vi "Test Initialization.vi"() -> ()   [LabVIEW 2015, in "String Compare Tests.lvlib"]
uses:
  String Compare Tests.lvlib
  classes/Sequence/Config/Sequence Config.lvclass
  Config/String Compare Config.lvclass
  <vilib>/NI/Tag Bus/tag/Data Type.ctl
  <vilib>/NI/Tag Bus Module Framework/channel/channel classification.ctl
  Config/Mode.ctl
  Config/String Compare Config.lvclass/String Compare Config.ctl
  Config/Write Test Value Channel.vi
  Config/Write Result Channel.vi
  Config/Write Mode.vi
  Config/Write Limit_Regex.vi
  Config/Write ignore case.vi
  Config/Write Multiline.vi
  Config/Write offset.vi
  classes/Sequence/Execution/Sequence.lvclass
  <vilib>/NI/Tag Bus Module Framework/channel/TBM channel.lvclass
  <vilib>/NI/Tag Bus/tag/tag descriptor.lvclass
panel:
  out "error out":errorcluster
  out "Pass":bool
  out "Name":string
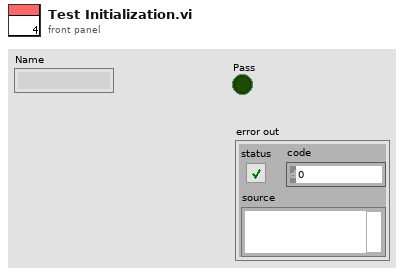
[diagram p1: front panel]
types:
  T1 = typedef "String Compare Config.lvclass/Mode.ctl" = enum16{"Compare Strings", "Match Regex"}
  T2 = typedef "TBM channel.lvclass/channel classification.ctl" = enum16{"input data", "output data", "processing parameter", "processing result"}
  T3 = typedef "tag bus.lvlib/tag descriptor.lvclass/Data Type.ctl" = enum16{"Double", "Single", "I64", "I32", "I16", "I8", "U64", "U32", "U16", "U8", "Boolean", "String", "Array of Double", "Array of Single", "Array of I64", "Array of I32", "Array of I16", "Array of I8", "Array of U64", "Array of U32", "Array of U16", "Array of U8", "Array of Boolean", "Array of String"}
  T4 = typedef "TBM channel.lvclass/data tables.ctl" = cluster{"input data":T5, "processing parameter":T5, "processing result":T5, "output data":T5}
  T5 = typedef "tag bus.lvlib/dictionary table pair.ctl" = cluster{"data dictionary":refnum<class "data dictionary.lvclass">, "data table":T6}
  T6 = typedef "tag bus.lvlib/data table.lvlib/data table.ctl" = cluster{"Double":dbl[], "Single":sgl[], "I64":i64[], "I32":i32[], "I16":i16[], "I8":i8[], "U64":u64[], "U32":u32[], "U16":u16[], "U8":u8[], "Boolean":bool[], "String":string[], "Array of Double":cluster{"DBL Array":dbl[]}[], "Array of Single":cluster{"SGL Array":sgl[]}[], "Array of I64":cluster{"I64 Array":i64[]}[], "Array of I32":cluster{"I32 Array":i32[]}[], "Array of I16":cluster{"I16 Array":i16[]}[], "Array of I8":cluster{"I8 Array":i8[]}[], "Array of U64":cluster{"U64 Array":u64[]}[], "Array of U32":cluster{"U32 Array":u32[]}[], "Array of U16":cluster{"U16 Array":u16[]}[], "Array of U8":cluster{"U8 Array":u8[]}[], "Array of Boolean":cluster{"Boolean Array":bool[]}[], "Array of String":cluster{"String Array":string[]}[]}
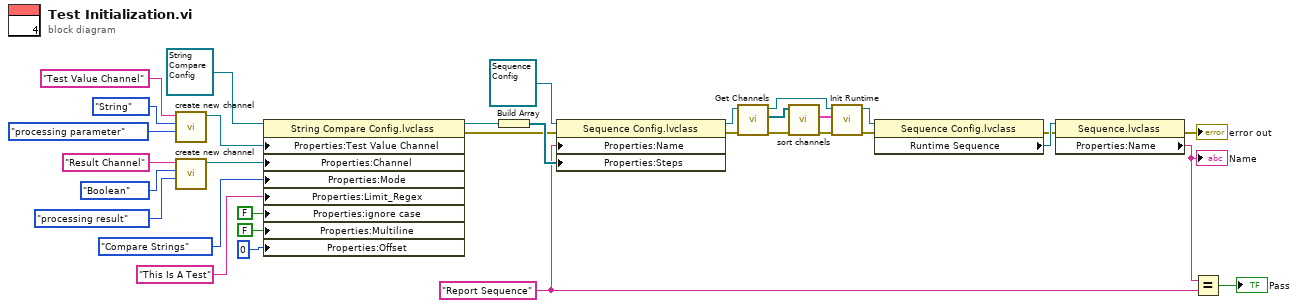
[diagram p0: block diagram]
diagram:
  w19 = "Report Sequence" ("Name")
  n1 = call <vilib>:"create new channel.vi"("channel classification"=channel_classification."processing parameter", "data type"=Data_Type."String", "channel name"="Test Value Channel") -> ("channel"=w9:refnum<class "TBM channel.lvclass">)  [unwired: 8 in]
  n2 = call <vilib>:"create new channel.vi"("channel classification"=channel_classification."processing result", "data type"=Data_Type."Boolean", "channel name"="Result Channel") -> ("channel"=w8:refnum<class "TBM channel.lvclass">)  [unwired: 8 in]
  n3 = property class="String Compare Config.lvclass"(reference=refnum<class "String Compare Config.lvclass"> refnum ("String Compare Config.lvclass"), "Properties:Test Value Channel"=w9, "Properties:Channel"=w8, "Properties:Mode"=Mode."Compare Strings" ("Mode"), "Properties:Limit_Regex"="This Is A Test" ("Limit_Regex"), "Properties:ignore case"=FALSE ("ignore case"), "Properties:Multiline"=FALSE ("Multiline"), "Properties:Offset"=0 ("Offset")) -> (reference out=w2:refnum<class "String Compare Config.lvclass">, error out=w1:errorcluster)  [unwired: 1 in]
  n4 = Build Array(w2) -> (w25:refnum<class "String Compare Config.lvclass">[])
  n5 = property class="Sequence Config.lvclass"(reference=refnum<class "Sequence Config.lvclass"> refnum ("Sequence Config.lvclass"), error in=w1, "Properties:Name"=w19, "Properties:Steps"=w25) -> (reference out=w24:refnum<class "Sequence Config.lvclass">, error out=w22:errorcluster)
  n6 = call "Get Channels.vi"("error in (no error)"=w22, "Sequence Config in"=w24) -> ("error out"=w30:errorcluster, "Channels"=w32:refnum<class "TBM channel.lvclass">[], "Sequence Config out"=w33:refnum<class "Sequence Config.lvclass">)  [unwired: 7 in]
  n7 = call <vilib>:"sort channels.vi"("error in"=w30, "channels in"=w32) -> ("error out"=w29:errorcluster, "data allocations"=w31:T4)  [unwired: 7 in, 1 out]
  n8 = call-dynamic "Init Runtime.vi"("error in (no error)"=w29, "data allocations"=w31, "Sequence Config in"=w33) -> ("error out"=w23:errorcluster, "Sequence Config out"=w28:refnum<class "Sequence Config.lvclass">)  [unwired: 7 in]
  n9 = property class="Sequence Config.lvclass"(reference=w28, error in=w23) -> (error out=w21:errorcluster, "Runtime Sequence"=w27:refnum<class "Sequence.lvclass">)  [unwired: 1 out]
  n10 = property class="Sequence.lvclass"(reference=w27, error in=w21) -> (error out=→"error out":errorcluster, "Properties:Name"=w20:string)  [unwired: 1 out]
  "Name" <- w20
  n11 = Equal?(x=w20, y=w19) -> (x = y?=→"Pass":bool)
